vi "OpenDB.vi"(8 "Error In":errorcluster, 9 "Password":string, 10 "Username":string, 11 "DB-Name":string) -> (0 "error out":errorcluster, 3 "connection reference":T1)   [LabVIEW 2017, in "Server.lvlib" / "Oracle.lvlib"]
uses:
  Oracle.lvlib
  <vilib>/addons/database/Connection.llb/Conn ObjectReference.ctl
  <vilib>/addons/database/Connection.llb/DB Tools Open Connec (String).vi
  <vilib>/addons/database/NI_Database_API.lvlib
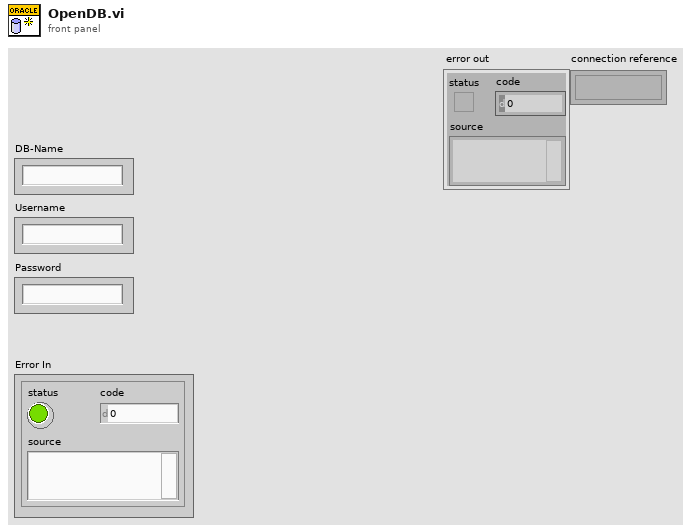
[diagram p1: front panel]
types:
  T1 = typedef "NI_Database_API.lvlib/Conn ObjectReference.ctl" = refnum<k1>
  T2 = typedef "NI_Database_API.lvlib/Conn DataMembers.ctl" = cluster{"ADODB._Connection":refnum<k7>, "recordset objects":i32, "command objects":i32}
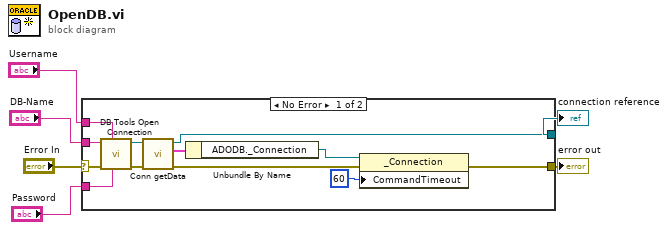
[diagram p0: block diagram]
diagram:
  n1 = case shown="No Error" "Error In" {
    selector: "Error In" -> [w8 w19]
    tunnel: "DB-Name" -> [w18 _]
    tunnel: "Username" -> [w17 _]
    tunnel: "Password" -> [w16 _]
    tunnel: [w7 w19] -> w3
    tunnel: [w9 _] -> w2
    frame No Error {
      n2 = call-poly <vilib>:"DB Tools Open Connection.vi"("password"=w16, "userID"=w17, "error in (no error)"=w8, "connection information"=w18) -> ("error out"=w11:errorcluster, "connection reference"=w10:T1)  [unwired: 4 in]
      n3 = call <vilib>:"Conn getData.vi"("error in (no error)"=w11, "connection reference"=w10) -> ("error out"=w13:errorcluster, "data"=w15:T2, "connection reference out"=w9:T1)  [unwired: 3 out]
      n4 = Unbundle By Name(w15) -> ("ADODB._Connection"=w12:refnum<k7>)
      n5 = property class="_Connection"(reference=w12, error in=w13, "CommandTimeout"=60) -> (error out=w7:errorcluster)  [unwired: 1 out]
    }
    frame Error {
    }
  }
  "error out" <- w3
  "connection reference" <- w2
